vi "file format.vi"(8 "error in (no error)":errorcluster, 10 "Tipo de archivo":enum16{"TXT", "BIN"}(ring) caption="Enum 3", 11 "GUI_Graph in":refnum<class "GUI_Graph.lvclass">) -> (0 "error out":errorcluster, 3 "GUI_Graph out":refnum<class "GUI_Graph.lvclass">)   [LabVIEW 2020, in "GUI_Graph.lvlib" / "GUI_Graph.lvclass"]
uses:
  GUI_Graph.lvclass
  C:/Program Files/National Instruments/LabVIEW 2020/vi.lib/ActorFramework/Actor/Actor.lvclass
  Loggin/Loggin/Loggin.lvclass
  Binary/Binary/Binary.lvclass
  C:/Users/Ceci Saldivar/Desktop/ceci/7mo semestre/Henry/Actor-Tarea-10-12-2020/Loggin/Loggin/Loggin.lvclass
  GUI_Graph.lvclass/GUI_Graph.ctl
  <vilib>/ActorFramework/Actor/Actor.lvclass
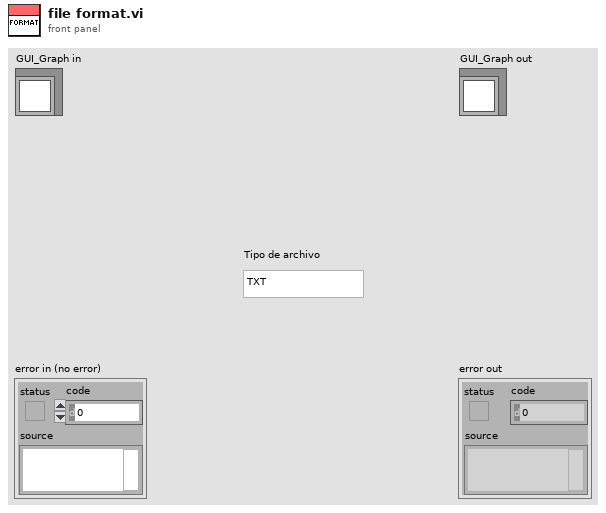
[diagram p1: front panel]
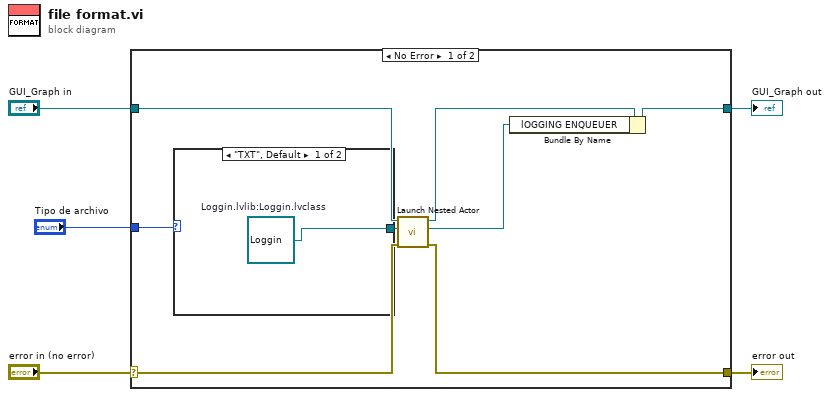
[diagram p0: block diagram]
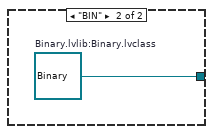
[diagram p2: hidden frame]
diagram:
  n1 = case shown="No Error" "error in (no error)" {
    selector: "error in (no error)" -> [w7 w17]
    tunnel: [w6 w17] -> w4
    tunnel: [w9 w16] -> w2
    tunnel: "GUI_Graph in" -> [w11 w16]
    tunnel: "Tipo de archivo" -> [w13 _]
    frame No Error {
      n2 = case shown="\"TXT\", Default" w13 {
        tunnel: [w14 w15] -> w12
        frame "TXT", Default {
          w14 = refnum<class "Loggin.lvclass"> refnum  # Loggin.lvlib:Loggin.lvclass
        }
        frame "BIN" {
          w15 = refnum<class "Binary.lvclass"> refnum  # Binary.lvlib:Binary.lvclass
        }
      }
      n3 = call <vilib>:"Launch Nested Actor.vi"("error in (no error)"=w7, "Nested Actor"=w12, "Caller Actor in"=w11) -> ("error out"=w6:errorcluster, "Nested Actor's Enqueuer"=w8:refnum<class "Message Enqueuer.lvclass">, "Caller Actor out"=w10:refnum<class "GUI_Graph.lvclass">)  [unwired: 6 in]
      n4 = Bundle By Name(cluster=w10, "lOGGING ENQUEUER"=w8) -> (w9:refnum<class "GUI_Graph.lvclass">)
    }
    frame Error {
    }
  }
  "error out" <- w4
  "GUI_Graph out" <- w2
